vi "display.length_in_pixels.vi"(8 "error in (no error)":errorcluster, 11 "midi-ui in":refnum<class "midi-ui.lvclass">) -> (0 "error out":errorcluster, 1 "White Key Length (px)":dbl, 2 "note board Length (px)":dbl, 3 "midi-ui out":refnum<class "midi-ui.lvclass">)   [LabVIEW 2020, in "midi-ui.lvclass"]
uses:
  midi-ui.lvclass
  midi-ui.lvclass/midi-ui.ctl
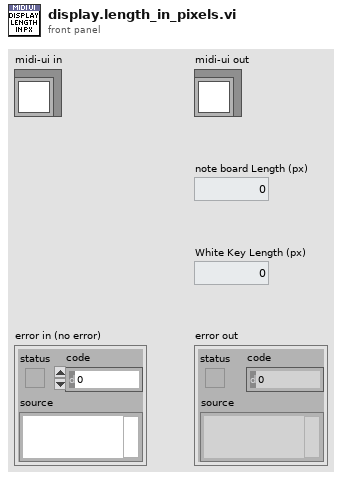
[diagram p1: front panel]
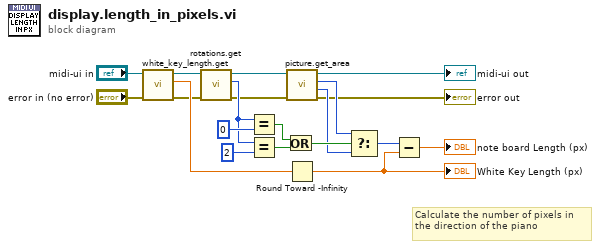
[diagram p0: block diagram]
diagram:
  # "Calculate the number of pixels in the direction of the piano"
  n1 = call "white_key_length.get.vi"("error in (no error)"="error in (no error)", "midi-ui in"="midi-ui in") -> ("error out"=w6:errorcluster, "White Key Length"=w11:dbl, "midi-ui out"=w5:refnum<class "midi-ui.lvclass">)  [unwired: 7 in]
  n2 = call "rotations.get.vi"("error in (no error)"=w6, "midi-ui in"=w5) -> ("error out"=w1:errorcluster, "Anticlockwise rotations [0-3] (0)"=w10:i32, "midi-ui out"=w4:refnum<class "midi-ui.lvclass">)  [unwired: 7 in]
  n3 = Equal?(x=w10, y=0) -> (x = y?=w18:bool)
  n4 = Equal?(x=w10, y=2) -> (x = y?=w17:bool)
  n5 = Or(x=w18, y=w17) -> (x .or. y?=w16:bool)
  n6 = call "picture.get_area.vi"("error in (no error)"=w1, "midi-ui in"=w4) -> ("error out"=→"error out":errorcluster, "Bounds:Area Width"=w12:u32, "Bounds:Area Height"=w13:u32, "midi-ui out"=→"midi-ui out":refnum<class "midi-ui.lvclass">)  [unwired: 6 in]
  n7 = Round Toward -Infinity(1:w11) -> (0:w14:dbl)
  "White Key Length (px)" <- w14
  n8 = Select(t=w13, s=w16, f=w12) -> (s? t:f=w15:u32)
  n9 = Subtract(x=w15, y=w14) -> (x-y=→"note board Length (px)":dbl)
